vi "test_equipo.vi"() -> ()   [LabVIEW 2019, in "Pistofono.lvclass"]
uses:
  Pistofono.lvclass
panel:
  out "code":i32
  out "opcion2":i32
  out "opcion1":i32
  out "hPa":dbl
  out "dB":dbl
  out "C":dbl
  in  "stop1":bool
  out "C":dbl
  in  "error in":errorcluster
  out "error out":errorcluster
  in  "stop2":bool
  in  "opciones":bool
  # "false = opcion 1\ntru = opcion 2"
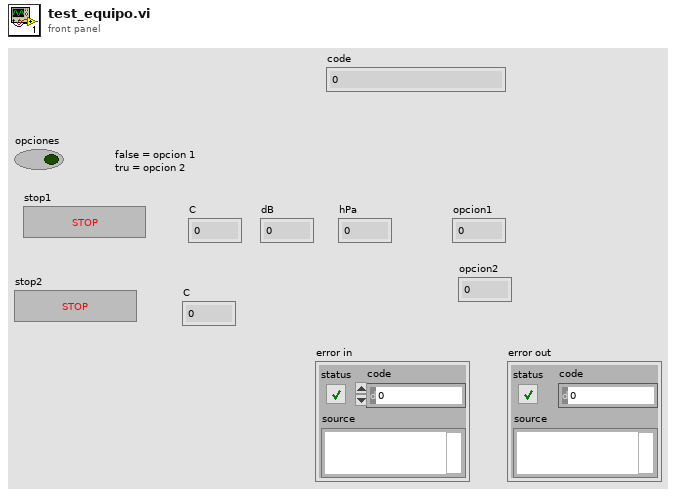
[diagram p1: front panel]
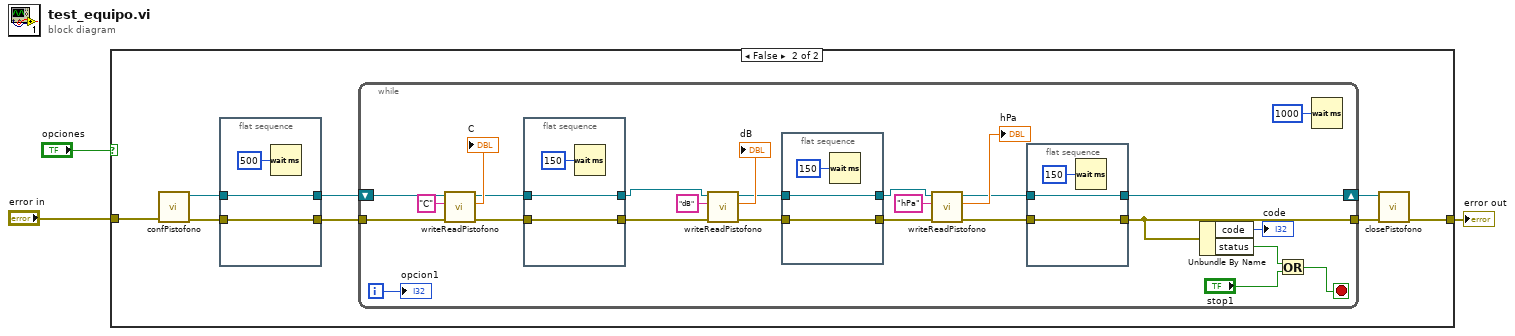
[diagram p0: block diagram]
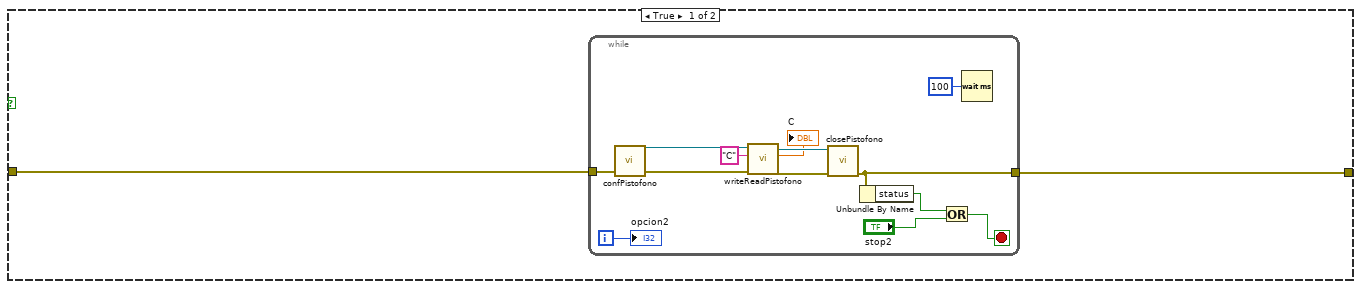
[diagram p2: hidden frame]
diagram:
  n1 = case shown="False" "opciones" {
    tunnel: [w5 w24] -> w2
    tunnel: "error in" -> [w4 w23]
    frame True {
      n2 = while {
        tunnel: [w15] -> w5
        tunnel: w4 -> [w14]
        i -> [w7]
        stop <- w17 stop-if-true
        n3 = call "confPistofono.vi"("error in (no error)"=w14) -> ("error out"=w12:errorcluster, "Pistofono out"=w13:refnum<class "Pistofono.lvclass">)  [unwired: 8 in, 1 out]
        n4 = call "writeReadPistofono.vi"("error in (no error)"=w12, "Command"="C", "Pistofono in"=w13) -> ("error out"=w10:errorcluster, "medicion (num)"=→"C":dbl, "Pistofono out"=w11:refnum<class "Pistofono.lvclass">)  [unwired: 6 in]
        n5 = call "closePistofono.vi"("error in (no error)"=w10, "Pistofono in"=w11) -> ("error out"=w15:errorcluster)  [unwired: 8 in, 1 out]
        n6 = Unbundle By Name(w15) -> ("status"=w18:bool)
        n7 = Or(x=w18, y="stop2") -> (x .or. y?=w17:bool)
        n8 = Wait (ms)(milliseconds to wait=u32 100) -> ()  [unwired: 1 out]
        "opcion2" <- w7
      }
    }
    frame False {
      n9 = call "confPistofono.vi"("error in (no error)"=w23) -> ("error out"=w22:errorcluster, "Pistofono out"=w21:refnum<class "Pistofono.lvclass">)  [unwired: 8 in, 1 out]
      n10 = flat-sequence {
        tunnel: w22 -> [w29]
        tunnel: [w29] -> w20
        tunnel: [w28] -> w19
        tunnel: w21 -> [w28]
        frame #0 {
          n11 = Wait (ms)(milliseconds to wait=u32 500) -> ()  [unwired: 1 out]
        }
      }
      n12 = while {
        tunnel: w20 -> [w55]
        tunnel: [w38] -> w25
        shift-right: [w32] -> w26
        shift-left: w19 -> [w51]
        i -> [w44]
        stop <- w52 stop-if-true
        n13 = call "writeReadPistofono.vi"("error in (no error)"=w55, "Command"="C", "Pistofono in"=w51) -> ("error out"=w41:errorcluster, "medicion (num)"=→"C":dbl, "Pistofono out"=w37:refnum<class "Pistofono.lvclass">)  [unwired: 6 in]
        n14 = flat-sequence {
          tunnel: w41 -> [w64]
          tunnel: [w64] -> w40
          tunnel: [w63] -> w36
          tunnel: w37 -> [w63]
          frame #0 {
            n15 = Wait (ms)(milliseconds to wait=u32 150) -> ()  [unwired: 1 out]
          }
        }
        n16 = call "writeReadPistofono.vi"("error in (no error)"=w40, "Command"="dB", "Pistofono in"=w36) -> ("error out"=w42:errorcluster, "medicion (num)"=→"dB":dbl, "Pistofono out"=w35:refnum<class "Pistofono.lvclass">)  [unwired: 6 in]
        n17 = flat-sequence {
          tunnel: w42 -> [w61]
          tunnel: [w61] -> w39
          tunnel: [w60] -> w34
          tunnel: w35 -> [w60]
          frame #0 {
            n18 = Wait (ms)(milliseconds to wait=u32 150) -> ()  [unwired: 1 out]
          }
        }
        n19 = call "writeReadPistofono.vi"("error in (no error)"=w39, "Command"="hPa", "Pistofono in"=w34) -> ("error out"=w43:errorcluster, "medicion (num)"=→"hPa":dbl, "Pistofono out"=w33:refnum<class "Pistofono.lvclass">)  [unwired: 6 in]
        n20 = flat-sequence {
          tunnel: w43 -> [w58]
          tunnel: [w58] -> w38
          tunnel: w33 -> [w57]
          tunnel: [w57] -> w32
          frame #0 {
            n21 = Wait (ms)(milliseconds to wait=u32 150) -> ()  [unwired: 1 out]
          }
        }
        n22 = Unbundle By Name(w38) -> ("code"=→"code":i32, "status"=w54:bool)
        n23 = Or(x=w54, y="stop1") -> (x .or. y?=w52:bool)
        n24 = Wait (ms)(milliseconds to wait=u32 1000) -> ()  [unwired: 1 out]
        "opcion1" <- w44
      }
      n25 = call "closePistofono.vi"("error in (no error)"=w25, "Pistofono in"=w26) -> ("error out"=w24:errorcluster)  [unwired: 8 in, 1 out]
    }
  }
  "error out" <- w2
